vi "Vision Research Phantom Series PhCon PhNVMContRec.vi"(0 "CN in":u32=1, 2 "pEnable":T1, 5 "Error In (no error)":errorcluster) -> (14 "CN out":u32=1, 16 "pSave":bool, 17 "pOldValue":u32, 19 "Error Out":errorcluster)   [LabVIEW 2013, in "VRI.lvlib"]
doc: "PhCon.dll\n\nPhNVMContRec\nHRESULT PhNVMContRec (UINT CN, PBOOL pSave, PUINT pOldValue,PUINT pEnable)\n\nParameters Description\nCN (in) Camera number\npSave (out) Camera is saving the cine to the NVM or is automaticall playing back to video\n pOldValue (out) return the old status\npEnable (in) Enable or disable the continuous recording mode\n (0=disable 1=enable 3=enable Cont Rec with automatic playback)\nReturn HRESULT (0=Ok)\nComments Set the continuous recording mode for the nonvolatile memory:\n When a cine is available it is saved in the NV memory and the recording of \n a new cine is automatically started Test if a cine save to NVM operation is \n in progress using the pSave.\n Any pointer can be NULL.\n\nWritten by:\nBLOOMY CONTROLS, INC\nWINDSOR, CT 06095, USA\n860-298-9925\nwww.bloomy.com\nV1.0.0\nMay, 2004"
uses:
  VRI.lvlib
  _Type Defs/pEnable.ctl
  Phantom DLLs/PhCon.dll
panel:
  # "For instructions on the use of this VI, press Ctrl+H to display the help window and move the mouse over the icon, controls, and indicators"
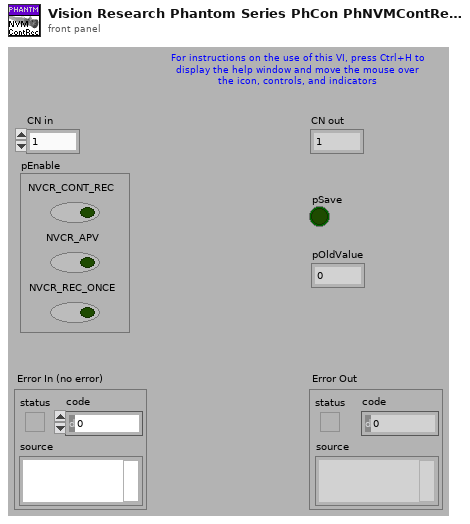
[diagram p1: front panel]
types:
  T1 = typedef "VRI.lvlib/pEnable.ctl" = cluster{"NVCR_CONT_REC":bool, "NVCR_APV":bool, "NVCR_REC_ONCE":bool}
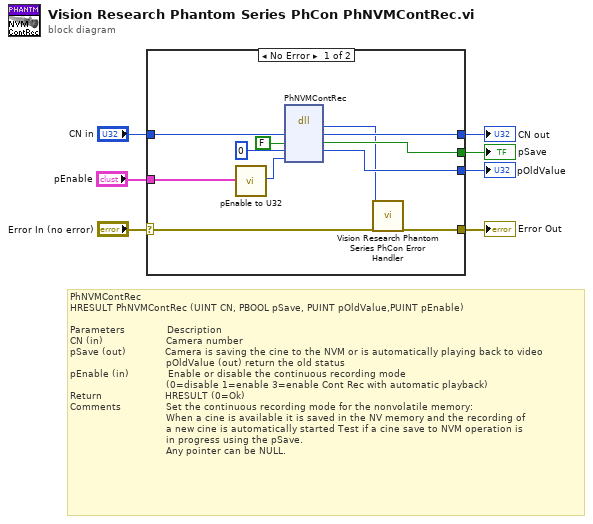
[diagram p0: block diagram]
diagram:
  # "PhNVMContRec\nHRESULT PhNVMContRec (UINT CN, PBOOL pSave, PUINT pOldValue,PUINT pEnable)\n\nParameters              Description\nCN (in)                     Camera number\npSave (out)             Camera is saving the cine to the NVM or is automatically playing back to video\n                                pOldValue (out) return the old status\npEnable (in)             Enable or disable the continuous recording mode\n                                (0=disable 1=enable 3=enable Cont Rec with automatic playback)\nReturn                     HRESULT (0=Ok)\nComments               Set the continuous recording mode for the nonvolatile memory:\n                                When a cine is available it is saved in the NV memory and the recording of \n                                a new cine is automatically started Test if a cine save to NVM operation is \n                                in progress using the pSave.\n                                Any pointer can be NULL."
  n1 = case shown="No Error" "Error In (no error)" {
    selector: "Error In (no error)" -> [w18 w20]
    tunnel: [w17 w20] -> w6
    tunnel: "CN in" -> [w16 w19]
    tunnel: [w15 w19] -> w4
    tunnel: [w14 _] -> w3
    tunnel: [w13 _] -> w2
    tunnel: "pEnable" -> [w12 _]
    frame No Error {
      n2 = call "pEnable to U32.vi"("pEnable"=w12) -> ("pEnable out"=w8:u32)  [unwired: 18 out]
      n3 = dll-call lib="C:/Projects/SDK/32-bit/Vision Research Phantom Series Labview Driver/Phantom DLLs/PhCon.dll" fn="PhNVMContRec"("CN"=w16, FALSE, "pOldValue"=u32 0, "pEnable"=w8) -> ("HRESULT"=w11:i32, "CN"=w15:u32, w14:bool, "pOldValue"=w13:u32)  [unwired: 4 in, 2 out]
      n4 = call "Vision Research Phantom Series PhCon Error Handler.vi"("ErrNo"=w11, "Error In (no error)"=w18) -> ("Error Out"=w17:errorcluster)  [unwired: 17 out]
    }
    frame Error {
    }
  }
  "Error Out" <- w6
  "CN out" <- w4
  "pSave" <- w3
  "pOldValue" <- w2
